vi "Galvos um to Volts.vi"(1 "Image Size (um)":dbl) -> (0 "Voltage (V)":dbl)   [LabVIEW 2014]
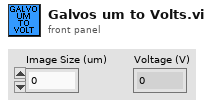
[diagram p1: front panel]
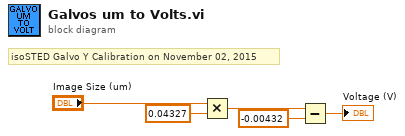
[diagram p0: block diagram]
diagram:
  # "isoSTED Galvo Y Calibration on November 02, 2015"
  n1 = Multiply(x="Image Size (um)", y=0.04327) -> (x*y=w4:dbl)
  n2 = Subtract(x=w4, y=-0.00432) -> (x-y=→"Voltage (V)":dbl)
